vi "StreamTransmitInstrumentGS.vi"() -> ()   [LabVIEW 2018]
panel:
  in  "Cluster":T1
  in  "stop 2":bool
  out "error out":errorcluster
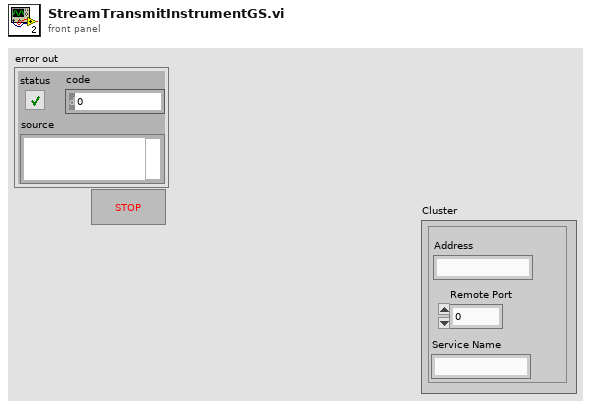
[diagram p1: front panel]
types:
  T1 = cluster{"Address":string, "Remote Port":u32, "Service Name":string}
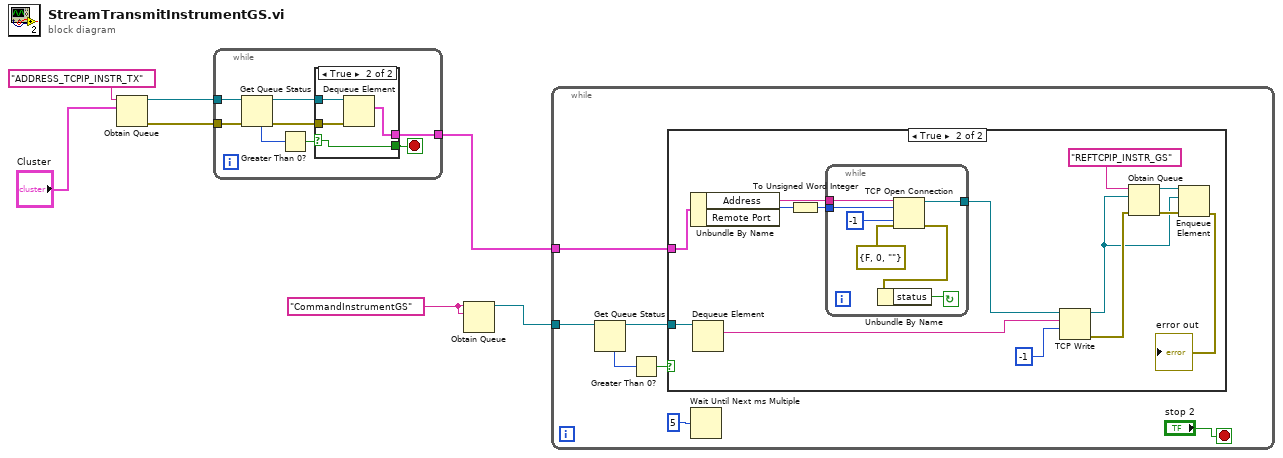
[diagram p0: block diagram]
diagram:
  w6 = "CommandInstrumentGS"
  n1 = Obtain Queue(name (unnamed)="ADDRESS_TCPIP_INSTR_TX", element data type="Cluster") -> (queue out=w2:refnum<queue>, error out=w3:errorcluster)  [unwired: 3 in, 1 out]
  n2 = while {
    tunnel: [w15] -> w4
    tunnel: w3 -> [w13]
    tunnel: w2 -> [w12]
    stop <- w8 stop-if-true
    n3 = Get Queue Status(queue=w12, error in (no error)=w13) -> (queue out=w11:refnum<queue>, error out=w14:errorcluster, # elements in queue=w10:i32)  [unwired: 1 in, 5 out]
    n4 = Greater Than 0?(x=w10) -> (x > 0?=w9:bool)
    n5 = case shown="True" w9 {
      selector: w9 -> [w16 w17]
      tunnel: [_ w20] -> w15
      tunnel: w14 -> [_ w19]
      tunnel: w11 -> [_ w18]
      tunnel: [w16 w17] -> w8
      frame False {
      }
      frame True {
        n6 = Dequeue Element(queue=w18, error in (no error)=w19) -> (element=w20:T1)  [unwired: 1 in, 3 out]
      }
    }
  }
  n7 = Obtain Queue(name (unnamed)=w6, element data type=w6) -> (queue out=w7:refnum<queue>)  [unwired: 3 in, 2 out]
  n8 = while {
    tunnel: w7 -> [w26]
    tunnel: w4 -> [w21]
    stop <- "stop 2" stop-if-true
    n9 = Get Queue Status(queue=w26) -> (queue out=w23:refnum<queue>, # elements in queue=w25:i32)  [unwired: 2 in, 6 out]
    n10 = Greater Than 0?(x=w25) -> (x > 0?=w24:bool)
    n11 = case shown="True" w24 {
      tunnel: w23 -> [_ w41]
      tunnel: w21 -> [_ w39]
      frame False {
      }
      frame True {
        n12 = Unbundle By Name(w39) -> ("Address"=w29:string, "Remote Port"=w28:u32)
        n13 = Dequeue Element(queue=w41) -> (element=w40:string)  [unwired: 2 in, 3 out]
        n14 = To Unsigned Word Integer(number=w28) -> (unsigned 16bit integer=w30:u16)
        n15 = while {
          tunnel: [w48] -> w38
          tunnel: w30 -> [w47]
          tunnel: w29 -> [w46]
          stop <- w42 continue-if-true
          n16 = TCP Open Connection(address=w46, remote port or service name=w47, timeout ms (60000)=-1, error in (no error)=errorcluster {"status"=FALSE, "code"=0, "source"=""}) -> (connection ID=w48:refnum<k5>, error out=w43:errorcluster)  [unwired: 1 in]
          n17 = Unbundle By Name(w43) -> ("status"=w42:bool)
        }
        n18 = TCP Write(connection ID=w38, data in=w40, 9:-1 ("timeout ms (25000)")) -> (connection ID out=w34:refnum<k5>, error out=w36:errorcluster)  [unwired: 1 in, 1 out]
        n19 = Obtain Queue(name (unnamed)="REFTCPIP_INSTR_GS", element data type=w34, error in (no error)=w36) -> (queue out=w33:refnum<queue>, error out=w35:errorcluster)  [unwired: 2 in, 1 out]
        n20 = Enqueue Element(queue=w33, element=w34, error in (no error)=w35) -> (error out=→"error out":errorcluster)  [unwired: 1 in, 2 out]
      }
    }
    n21 = Wait Until Next ms Multiple(millisecond multiple=u32 5) -> ()  [unwired: 1 out]
  }
